vi "Read Measurement (Channel Power).vi"(0 "VISA resource name":refnum<visa-resource-name>, 5 "Maximum Time (120000 ms)":i32=120000, 11 "error in (no error)":errorcluster) -> (4 "VISA resource name out":refnum<visa-resource-name>, 6 "Channel Power(dBm/Integrated BW MHz)":dbl, 10 "Channel Power Density(dBm/Hz)":dbl, 15 "error out":errorcluster)   [LabVIEW 2022 SP3, in "Agilent N934X Series.lvlib"]
doc: "Reads the measurement result from the spectrum analyzer(Channel Power Measurement)."
uses:
  <instrlib>/Agilent N934X Series/Agilent N934X Series.lvlib
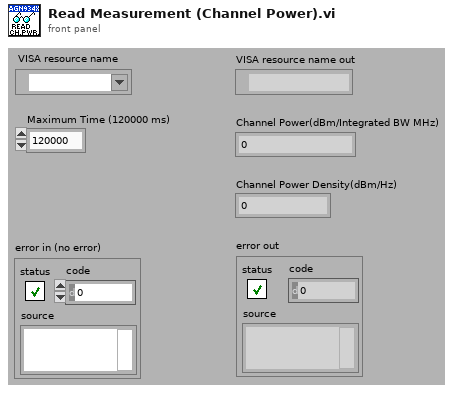
[diagram p1: front panel]
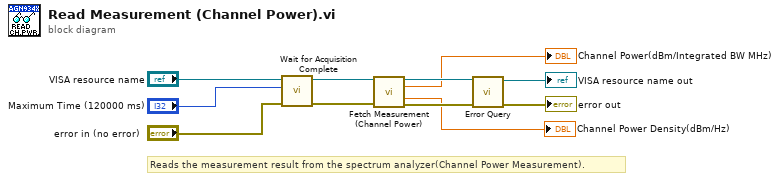
[diagram p0: block diagram]
diagram:
  # "Reads the measurement result from the spectrum analyzer(Channel Power Measurement)."
  n1 = call <instrlib>:"Wait for Acquisition Complete.vi"("error in (no error)"="error in (no error)", "Maximum Time (10000 ms)"="Maximum Time (120000 ms)", "VISA resource name"="VISA resource name") -> ("error out"=w10:errorcluster, "VISA resource name out"=w11:refnum<visa-resource-name>)  [unwired: 7 in]
  n2 = call <instrlib>:"Fetch Measurement (Channel Power).vi"("VISA resource name"=w11, "error in (no error)"=w10) -> ("VISA resource name out"=w6:refnum<visa-resource-name>, "Channel Power(dBm/Integrated BW MHz)"=→"Channel Power(dBm/Integrated BW MHz)":dbl, "Channel Power Density(dBm/Hz)"=→"Channel Power Density(dBm/Hz)":dbl, "error out"=w5:errorcluster)  [unwired: 10 in]
  n3 = call <instrlib>:"Error Query.vi"("error in (no error)"=w5, "VISA resource name"=w6) -> ("error out"=→"error out":errorcluster, "VISA resource name out"=→"VISA resource name out":refnum<visa-resource-name>)  [unwired: 6 in, 2 out]
